vi "mWmotor_get_ALARM.vi"(8 "error in (no error)":errorcluster, 10 "milliseconds to wait":u32=100, 11 "VISA resource name":refnum<visa-resource-name>) -> (0 "error out":errorcluster, 2 "Alarm code":i32, 3 "VISA resource name out":refnum<visa-resource-name>)   [LabVIEW 2019]
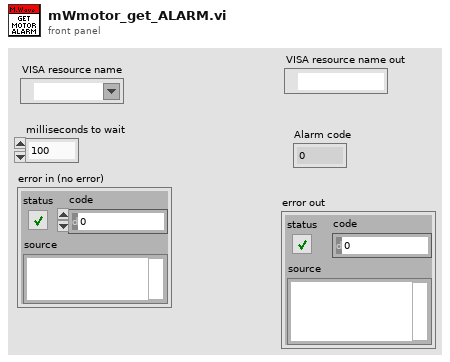
[diagram p1: front panel]
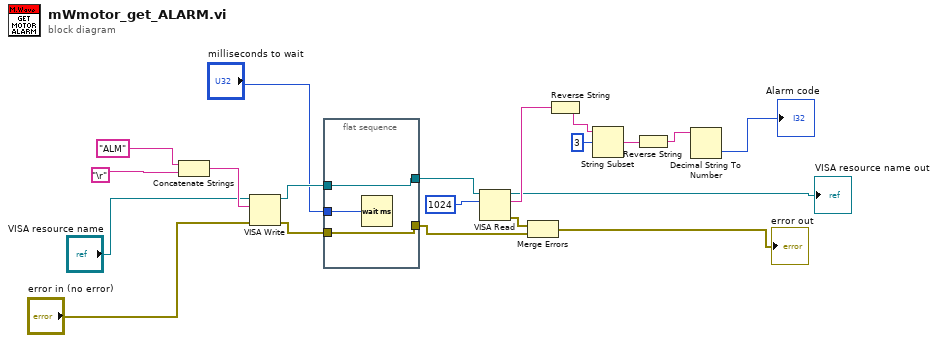
[diagram p0: block diagram]
diagram:
  n1 = Concatenate Strings("ALM" ("string"), "\r") -> (w20:string)
  n2 = VISA Write(VISA resource name="VISA resource name", write buffer=w20, error in (no error)="error in (no error)") -> (VISA resource name out=w16:refnum<visa-resource-name>, error out=w17:errorcluster)  [unwired: 1 out]
  n3 = flat-sequence {
    tunnel: [w23] -> w11
    tunnel: w17 -> [w23]
    tunnel: [w22] -> w15
    tunnel: w16 -> [w22]
    tunnel: "milliseconds to wait" -> [w21]
    frame #0 {
      n4 = Wait (ms)(milliseconds to wait=w21) -> ()  [unwired: 1 out]
    }
  }
  n5 = VISA Read(VISA resource name=w15, byte count=u32 1024) -> (VISA resource name out=→"VISA resource name out":refnum<visa-resource-name>, read buffer=w9:string, error out=w10:errorcluster)  [unwired: 1 in, 1 out]
  n6 = Merge Errors(w10, w11) -> (→"error out":errorcluster)
  n7 = Reverse String(1:w9) -> (0:w7:string)
  n8 = String Subset(string=w7, offset (0)=3) -> (substring=w6:string)  [unwired: 1 in]
  n9 = Reverse String(1:w6) -> (0:w5:string)
  n10 = Decimal String To Number(string=w5) -> (number=→"Alarm code":i32)  [unwired: 2 in, 1 out]
